vi "CSM_Project_Item_Interface.vi"() -> (3 "InterfaceTable":T1)   [LabVIEW 2017]
uses:
  <resource>/Framework/Providers/API/Item_Interface.ctl
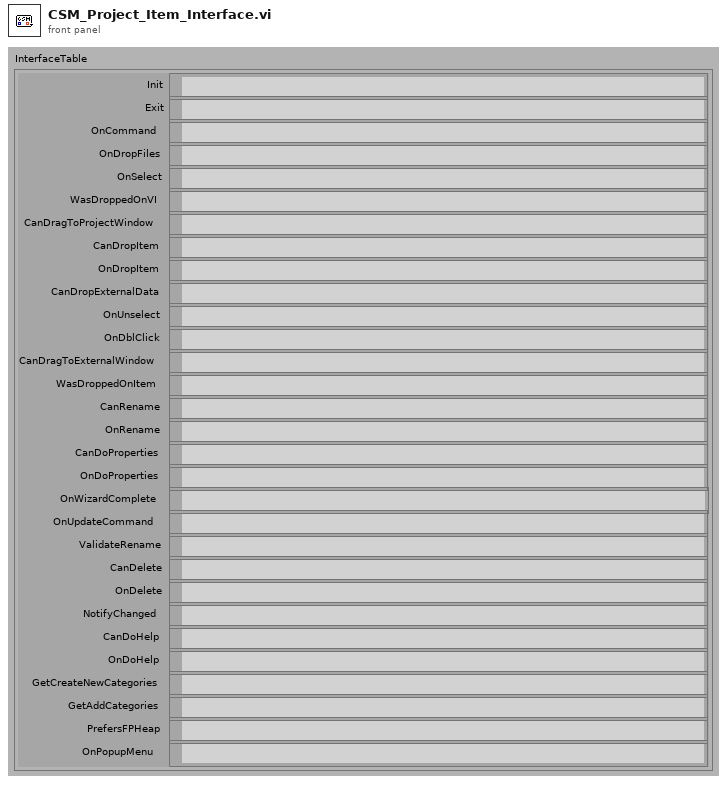
[diagram p1: front panel]
types:
  T1 = typedef "Item_Interface.ctl" = cluster{"Init":path, "Exit":path, "OnCommand":path, "OnDropFiles":path, "OnSelect":path, "WasDroppedOnVI":path, "CanDragToProjectWindow":path, "CanDropItem":path, "OnDropItem":path, "CanDropExternalData":path, "OnUnselect":path, "OnDblClick":path, "CanDragToExternalWindow":path, "WasDroppedOnItem":path, "CanRename":path, "OnRename":path, "CanDoProperties":path, "OnDoProperties":path, "OnWizardComplete":path, "OnUpdateCommand":path, "ValidateRename":path, "CanDelete":path, "OnDelete":path, "NotifyChanged":path, "CanDoHelp":path, "OnDoHelp":path, "GetCreateNewCategories":path, "GetAddCategories":path, "PrefersFPHeap":path, "OnPopupMenu":path}
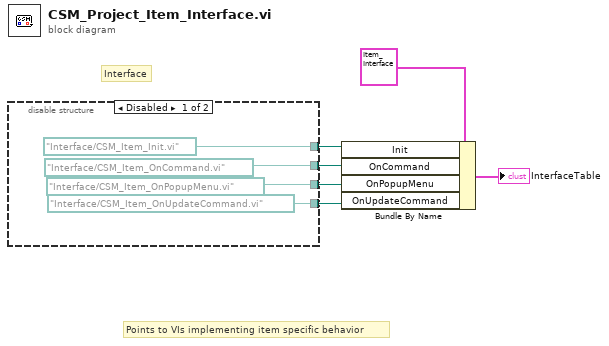
[diagram p0: block diagram]
diagram:
  # "Interface"
  # "Points to VIs implementing item specific behavior"
  n1 = disable-structure shown="Disabled" {
    disable-tunnel: [path "Interface/CSM_Item_Init.vi" ("Init") _] -> w4
    disable-tunnel: [path "Interface/CSM_Item_OnCommand.vi" ("OnCommand") _] -> w3
    disable-tunnel: [path "Interface/CSM_Item_OnPopupMenu.vi" ("OnPopupMenu") _] -> w2
    disable-tunnel: [path "Interface/CSM_Item_OnUpdateCommand.vi" ("OnPopupMenu") _] -> w1
    frame Disabled {
    }
    frame Enabled {
    }
  }
  n2 = Bundle By Name(cluster=T1 {"Init"=path "", "Exit"=path "", "OnCommand"=path "", "OnDropFiles"=path "", "OnSelect"=path "", "WasDroppedOnVI"=path "", "CanDragToProjectWindow"=path "", "CanDropItem"=path "", "OnDropItem"=path "", "CanDropExternalData"=path "", "OnUnselect"=path "", "OnDblClick"=path "", "CanDragToExternalWindow"=path "", "WasDroppedOnItem"=path "", "CanRename"=path "", "OnRename"=path "", "CanDoProperties"=path "", "OnDoProperties"=path "", "OnWizardComplete"=path "", "OnUpdateCommand"=path "", "ValidateRename"=path "", "CanDelete"=path "", "OnDelete"=path "", "NotifyChanged"=path "", "CanDoHelp"=path "", "OnDoHelp"=path "", "GetCreateNewCategories"=path "", "GetAddCategories"=path "", "PrefersFPHeap"=path "", "OnPopupMenu"=path ""} ("InterfaceTable"), "Init"=w4, "OnCommand"=w3, "OnPopupMenu"=w2, "OnUpdateCommand"=w1) -> (→"InterfaceTable":T1)
